vi "GetId.vi"(8 "error in":errorcluster, 11 "FailureReference in":refnum<class "FailureReference.lvclass">) -> (0 "error out":errorcluster, 2 "Id":string, 3 "FailureReference out":refnum<class "FailureReference.lvclass">)   [LabVIEW 2021, in "ProligentXMLGenerator.lvlib" / "FailureReference.lvclass"]
doc: "The identifier of the related failure."
uses:
  FailureReference.lvclass
  FailureReference.lvclass/FailureReference.ctl
  Base/Guid/Guid.lvclass
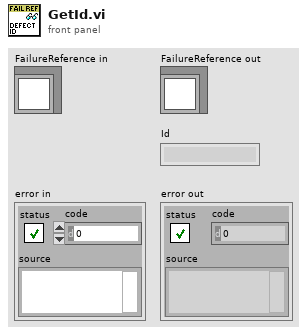
[diagram p1: front panel]
types:
  T1 = typedef "ProligentXMLGenerator.lvlib/FailureReference.lvclass/Data.ctl" = cluster{"Name":string, "CustomData":refnum<class "CustomData.lvclass">, "Id":refnum<class "Guid.lvclass">}
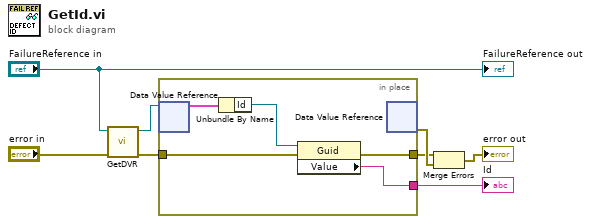
[diagram p0: block diagram]
diagram:
  n1 = call "GetDVR.vi"("error in"="error in", "FailureReference in"="FailureReference in") -> ("error out"=w4:errorcluster, "DVRReference"=w7:refnum<data-value>)  [unwired: 8 in]
  n2 = in-place "In Place Element Structure" {
    in-place-border: w4 -> [w11]
    in-place-border: [w10] -> w3
    in-place-border: [w9] -> w1
    n3 = in-place-dvr #1(w7) -> (w13:T1)  [unwired: 1 out]
    n4 = Unbundle By Name(w13) -> ("Id"=w12:refnum<class "Guid.lvclass">)
    n5 = property on="Property Node" class="Guid"(reference=w12, error in=w11) -> (error out=w10:errorcluster, "Value"=w9:string)  [unwired: 1 out]
    n6 = in-place-dvr #1() -> (w8:errorcluster)  [unwired: 1 in, 1 out]
  }
  "Id" <- w1
  n7 = Merge Errors(w3, w8) -> (→"error out":errorcluster)
  "FailureReference out" <- "FailureReference in"
